vi "Eval Multi-Variable Scalar.vi"(2 "error in (no error)":errorcluster, 3 "Variables":string[](array[string]), 4 "X Values":dbl[](array[numeric]) format="%.2f", 5 "formula":string) -> (0 "error out":errorcluster, 1 "y value":dbl format="%.2f")   [LabVIEW 2010, in "NI_Gmath.lvlib"]
doc: "Calculates exactly one function value based on a given formula."
uses:
  NI_Gmath.lvlib
panel:
  # "Example:\n\n formula: x*sin(y)\n X Values: (2.2,3.10)  \n Variables: x and y"
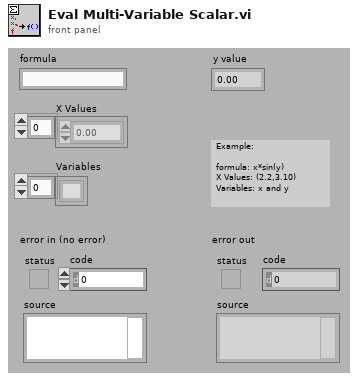
[diagram p1: front panel]
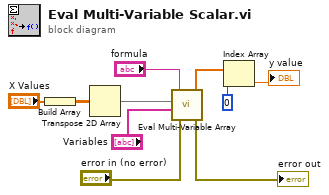
[diagram p0: block diagram]
diagram:
  n1 = Build Array("X Values") -> (w5:dbl[][])
  n2 = Transpose 2D Array(2D array=w5) -> (transposed array=w3:dbl[][])
  n3 = call "Eval Multi-Variable Array.vi"("error in (no error)"="error in (no error)", "Variables"="Variables", "X Values"=w3, "formula"="formula") -> ("error out"=→"error out":errorcluster, "Y Values"=w10:dbl[])
  n4 = Index Array(array=w10, index=0) -> (element=→"y value":dbl)
